vi "_Template.vi"(8 "error in (no error)":errorcluster, 11 "CommandLine":string[](array[string])) -> (0 "error out":errorcluster, 2 "test details":string)   [LabVIEW 2019]
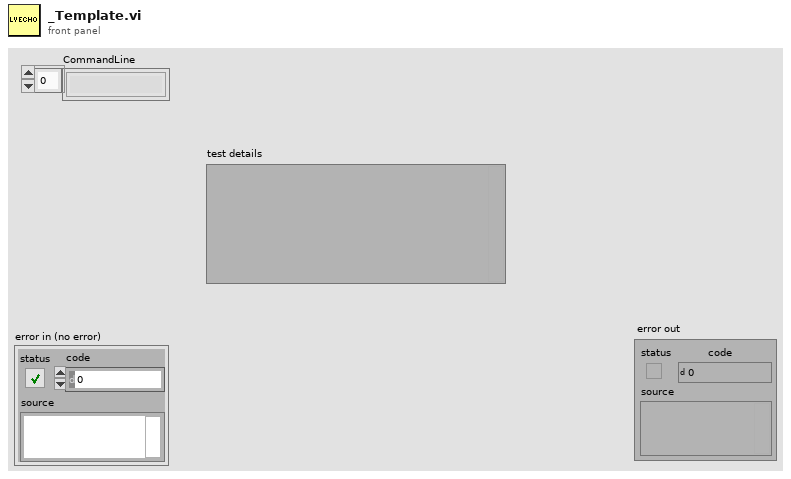
[diagram p1: front panel]
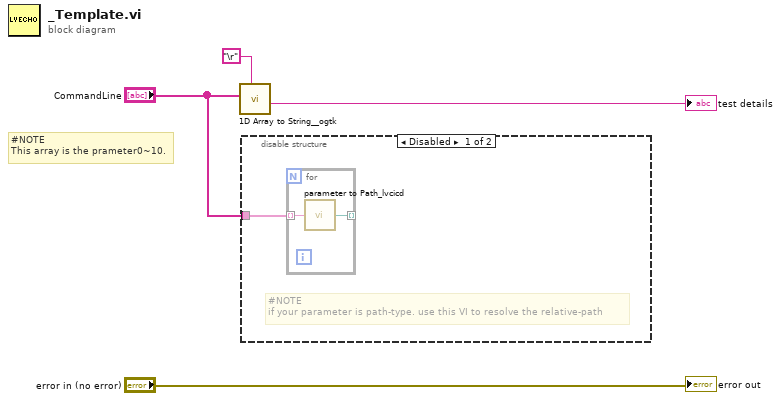
[diagram p0: block diagram]
diagram:
  # "#NOTE\nThis array is the prameter0~10."
  n1 = call <userlib>:"1D Array to String__ogtk.vi"("delimiter (Tab)"="\r", "Array of Strings"="CommandLine") -> ("delimited string"=→"test details":string)  [unwired: 9 in]
  n2 = disable-structure shown="Disabled" {
    disable-tunnel: "CommandLine" -> [w5 _]
    frame Disabled {
      # "#NOTE\nif your parameter is path-type. use this VI to resolve the relative-path"
      n3 = for {
        tunnel: [w7] -> _ mode=indexing
        tunnel: w5 -> [w6] mode=indexing
        n4 = call "parameter to Path_lvcicd.vi"("String"=w6) -> ("Path"=w7:path)
      }
    }
    frame Enabled {
    }
  }
  "error out" <- "error in (no error)"
